vi "RPC UI.vi"() -> ()   [LabVIEW 2015]
uses:
  <vilib>/NI/i3 JSON/JSON Generation/Create Value Files/Create Value - 1D Array Double.vi
  Classes/Server/Format Client Request (Numeric).vi
  Classes/Server/Send Request (Async).vi
  Classes/Server/Format Client Request (Auto-Increment).vi
  Classes/Server/Send Request (Sync).vi
  Classes/Server/JSONRPC Server.lvclass
  <vilib>/NI/i3 JSON/i3-json.lvlib
panel:
  in  "id":i32
  in  "B":dbl
  in  "A":dbl
  in  "stop":bool
  out "Response String":string
  out "found":bool
  in  "Check for Response":bool
  out "Response String":string
  in  "Send Sync Request":bool
  in  "Send Async Request":bool
  # "Subtraction"
  # "-"
  # "Asynchronous"
  # "Synchronous"
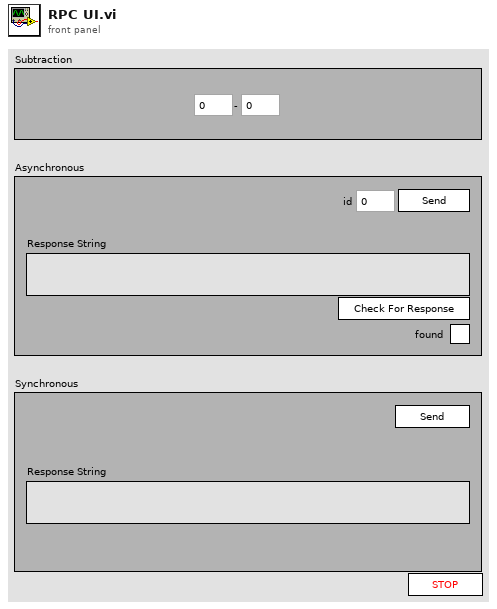
[diagram p1: front panel]
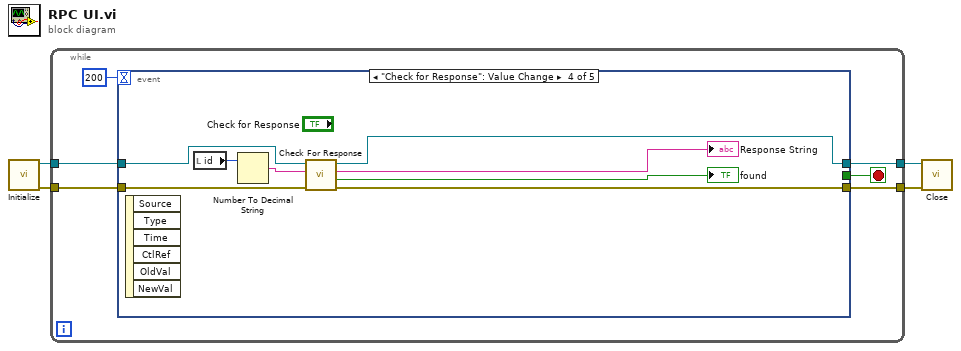
[diagram p0: block diagram]
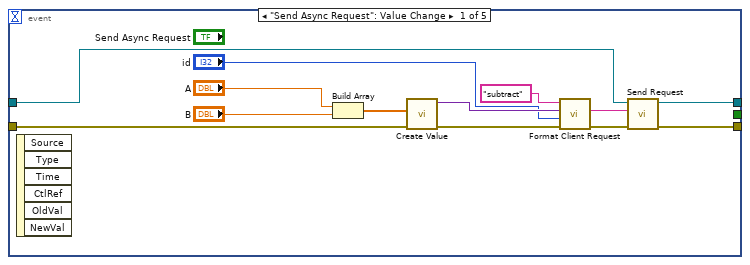
[diagram p2: hidden frame]
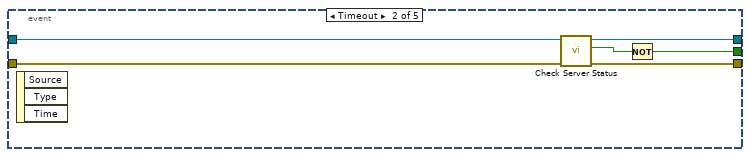
[diagram p3: hidden frame]
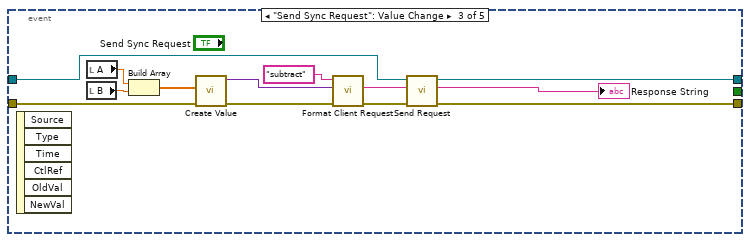
[diagram p4: hidden frame]
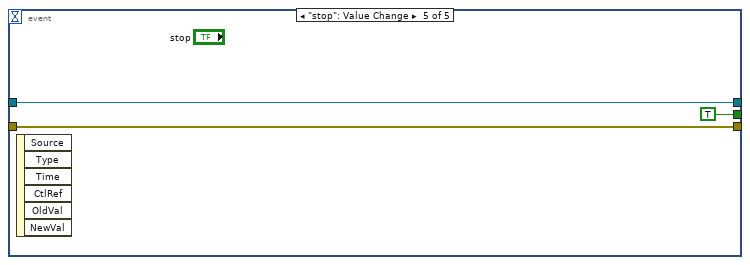
[diagram p5: hidden frame]
diagram:
  n1 = call "Initialize.vi"() -> ("error out"=w1:errorcluster, "Server Out"=w4:refnum<class "JSONRPC Server.lvclass">)  [unwired: 10 in]
  n2 = while {
    tunnel: w4 -> [w10]
    tunnel: [w8] -> w3
    tunnel: [w7] -> w2
    tunnel: w1 -> [w6]
    stop <- w9 stop-if-true
    n3 = event shown="[3] \"Check for Response\": Value Change" {
      selector: _ -> [_ _ _ _ _]
      dyn-events: _ -> [_ _ _ _ _]
      timeout: 200 -> [_ _ _ _ _]
      tunnel: w10 -> [w23 w29 w41 w48 w52]
      tunnel: [_ w26 _ _ TRUE] -> w9
      tunnel: [w22 w25 w42 w47 w52] -> w8
      tunnel: [w21 w24 w39 w46 w51] -> w7
      tunnel: w6 -> [w14 w28 w31 w45 w51]
      event "Send Async Request": Value Change {
        n4 = event-data() -> ()  [unwired: 1 in, 6 out]
        n5 = Build Array("A", "B") -> (w16:dbl[])
        n6 = call-poly <vilib>:"Create Value.vi"("error in (no error)"=w14, "1D Numeric"=w16) -> ("error out"=w13:errorcluster, "JSON Tree"=w15:variant)  [unwired: 8 in]
        n7 = call-poly "Format Client Request.vi"("error in (no error)"=w13, "id"="id", "params"=w15, "method"="subtract") -> ("error out"=w12:errorcluster, "Request String"=w20:string)  [unwired: 6 in]
        n8 = call-poly "Send Request.vi"("error in (no error)"=w12, "JSON Request String"=w20, "Server in"=w23) -> ("error out"=w21:errorcluster, "Server out"=w22:refnum<class "JSONRPC Server.lvclass">)  [unwired: 5 in, 2 out]
      }
      event Timeout {
        n9 = event-data() -> ()  [unwired: 1 in, 3 out]
        n10 = call "Check Server Status.vi"("error in (no error)"=w28, "Request in"=w29) -> ("error out"=w24:errorcluster, "Server Running?"=w27:bool, "Request out"=w25:refnum<class "JSONRPC Server.lvclass">)  [unwired: 7 in]
        n11 = Not(x=w27) -> (.not. x?=w26:bool)
      }
      event "Send Sync Request": Value Change {
        n12 = event-data() -> ()  [unwired: 1 in, 6 out]
        n13 = local read "A"() -> (w37:dbl)
        n14 = local read "B"() -> (w38:dbl)
        n15 = Build Array(w37, w38) -> (w35:dbl[])
        n16 = call-poly <vilib>:"Create Value.vi"("error in (no error)"=w31, "1D Numeric"=w35) -> ("error out"=w33:errorcluster, "JSON Tree"=w34:variant)  [unwired: 8 in]
        n17 = call-poly "Format Client Request.vi"("error in (no error)"=w33, "params"=w34, "method"="subtract") -> ("error out"=w30:errorcluster, "Request String"=w32:string)  [unwired: 7 in]
        n18 = call-poly "Send Request.vi"("error in (no error)"=w30, "JSON Request String"=w32, "JSONRPC Server in"=w41) -> ("error out"=w39:errorcluster, "JSON Response String"=→"Response String":string, "JSONRPC Server out"=w42:refnum<class "JSONRPC Server.lvclass">)  [unwired: 6 in]
      }
      event "Check for Response": Value Change {
        n19 = event-data() -> ()  [unwired: 1 in, 6 out]
        n20 = local read "id"() -> (w43:i32)
        n21 = Number To Decimal String(number=w43) -> (decimal integer string=w44:string)  [unwired: 1 in]
        n22 = call-dynamic "Check For Response.vi"("error in (no error)"=w45, "id String"=w44, "Server in"=w48) -> ("error out"=w46:errorcluster, "found"=→"found":bool, "JSON Response String"=→"Response String":string, "Server out"=w47:refnum<class "JSONRPC Server.lvclass">)  [unwired: 5 in]
      }
      event "stop": Value Change {
        n23 = event-data() -> ()  [unwired: 1 in, 6 out]
      }
    }
  }
  n24 = call-dynamic "Close.vi"("error in (no error)"=w2, "Server in"=w3) -> ()  [unwired: 9 in, 1 out]
